vi "Required Font-Scale (Text Draw Settings).vi"(4 "Thickness (Default: 1)":i32=1, 7 "Text Drawing Settings in (Default: Simplex)":T1={"OpenCV Font Face"=enum."FONT_HERSHEY_SIMPLEX", "Font Scale"=1.0}, 8 "error in (no error)":errorcluster, 11 "Required Text Height":u16) -> (0 "error out":errorcluster, 3 "Text Drawing Settings out":T1)   [LabVIEW 2020, in "image.lvlib"]
uses:
  image.lvlib
  Text Drawing Settings.ctl
  Font Face.ctl
  common/Module Path.vi
  <vilib>/Utility/error.llb/Error Cluster From Error Code.vi
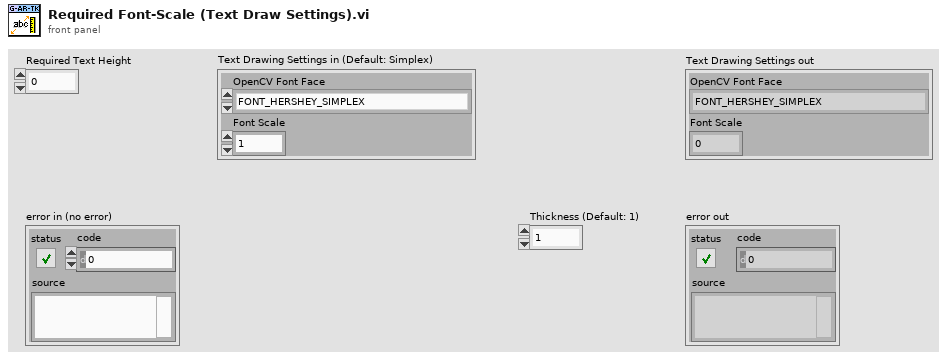
[diagram p1: front panel]
types:
  T1 = typedef "image.lvlib/Text Drawing Settings.ctl" = cluster{"OpenCV Font Face":T2, "Font Scale":dbl}
  T2 = typedef "image.lvlib/Font Face.ctl" = enum8{"FONT_HERSHEY_SIMPLEX", "FONT_HERSHEY_PLAIN", "FONT_HERSHEY_DUPLEX", "FONT_HERSHEY_COMPLEX", "FONT_HERSHEY_TRIPLEX", "FONT_HERSHEY_COMPLEX_SMALL", "FONT_HERSHEY_SCRIPT_SIMPLEX", "FONT_HERSHEY_SCRIPT_COMPLEX", "FONT_ITALIC"}
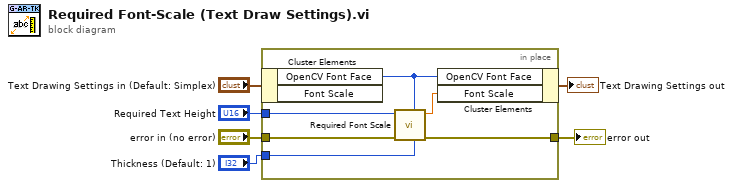
[diagram p0: block diagram]
diagram:
  n1 = in-place {
    in-place-border: "Required Text Height" -> [w12]
    in-place-border: "Thickness (Default: 1)" -> [w8]
    in-place-border: "error in (no error)" -> [w10]
    in-place-border: [w9] -> w2
    n2 = in-place-cluster #1("Text Drawing Settings in (Default: Simplex)") -> ("OpenCV Font Face"=w7:T2)  [unwired: 1 out]
    n3 = call "Required Font Scale.vi"("Thickness (Default: 1)"=w8, "OpenCV Font Face"=w7, "error in (no error)"=w10, "Required Text Height"=w12) -> ("error out"=w9:errorcluster, "Font Scale"=w11:dbl)  [unwired: 6 in]
    n4 = in-place-cluster #1("OpenCV Font Face"=w7, "Font Scale"=w11) -> (→"Text Drawing Settings out":T1)
  }
  "error out" <- w2
